vi "Read Continuous.vi"(8 "error In":errorcluster, 11 "Power Meter In":refnum<class "Power Meter.lvclass">) -> (0 "error out":errorcluster, 3 "Power Meter out":refnum<class "Power Meter.lvclass">)   [LabVIEW 2009, in "Power Meter.lvclass"]
doc: "A pop-up window for the Power Meter Control Panel that continuously reads the power until exited."
uses:
  Power Meter.lvclass
  Utility Classes/Readable/X.ctl
  Utility Classes/Readable/Readable.lvclass
panel:
  out "Power w/Units":string
  out "Power":T1
  in  "Read Continuous":bool
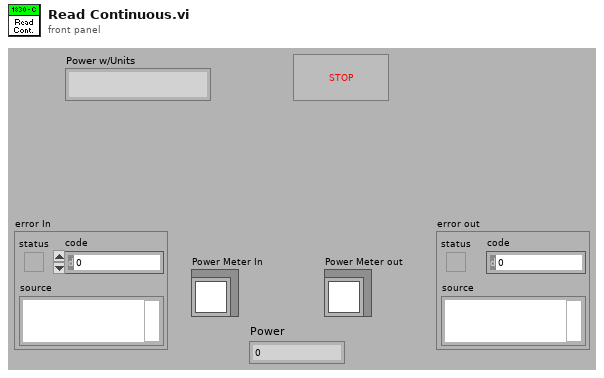
[diagram p1: front panel]
types:
  T1 = typedef "Readable.lvclass/X.ctl" = dbl
  T2 = typedef "Readable.lvclass/X array.ctl" = T1[]
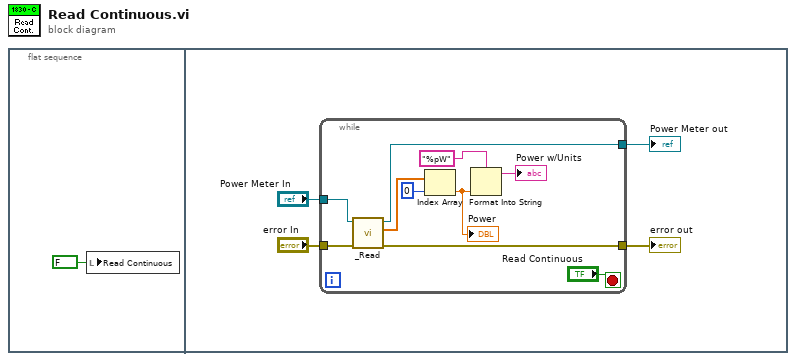
[diagram p0: block diagram]
diagram:
  n1 = flat-sequence {
    frame #0 {
      n2 = local write "Read Continuous"(FALSE ("Read Continuous")) -> ()
    }
    frame #1 {
      n3 = while {
        tunnel: "Power Meter In" -> [w12]
        tunnel: "error In" -> [w11]
        tunnel: [w10] -> w3
        tunnel: [w9] -> w2
        stop <- "Read Continuous" stop-if-true
        n4 = call-dynamic "_Read.vi"("error in (no error)"=w11, "Power Meter in"=w12) -> ("error out"=w9:errorcluster, "X array"=w15:T2, "Power Meter out"=w10:refnum<class "Power Meter.lvclass">)  [unwired: 7 in]
        n5 = Index Array(array=w15, index=0) -> (element=w6:T1)
        "Power" <- w6
        n6 = Format Into String(format string="%pW", w6) -> (resulting string=→"Power w/Units":string)  [unwired: 2 in, 1 out]
      }
      "Power Meter out" <- w3
      "error out" <- w2
    }
  }
